vi "REFPROPdll_Test.vi"(8 "error in (no error)":errorcluster) -> (0 "error out":errorcluster, 3 "Passed?":bool)   [LabVIEW 2016]
panel:
  out "Inputs":T1
  out "Outputs":T2
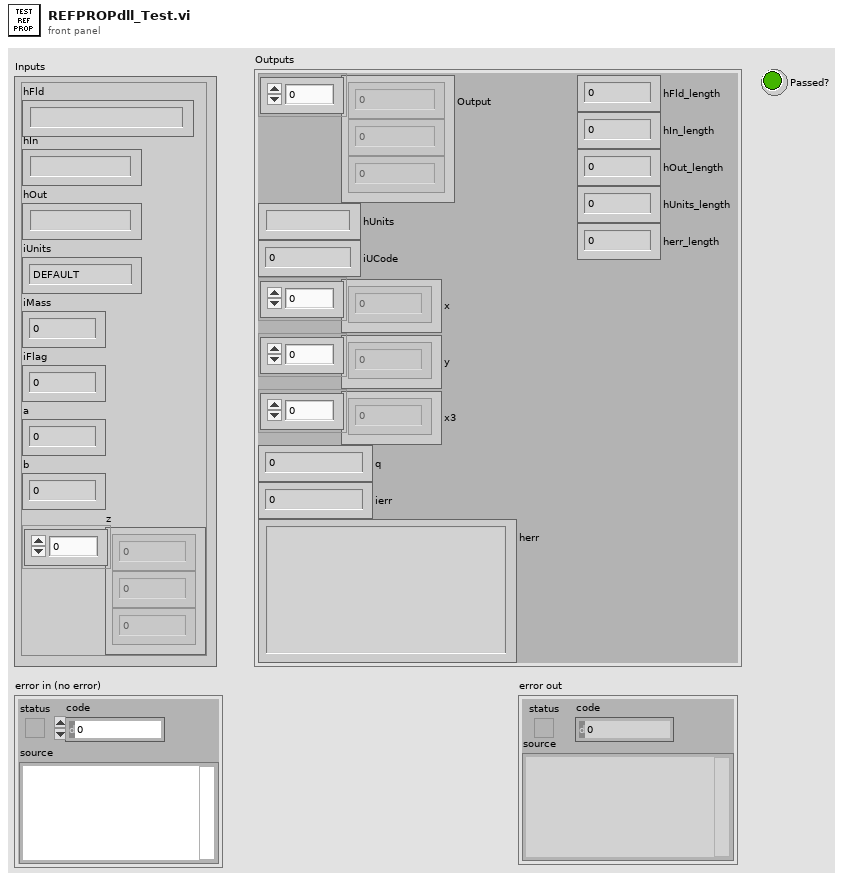
[diagram p1: front panel]
types:
  T1 = cluster{"hFld":string, "hIn":string, "hOut":string, "iUnits":enum32{"DEFAULT", "MOLE SI", "MASS SI", "SI WITH C"}, "iMass":i32, "iFlag":i32, "a":dbl, "b":dbl, "z":dbl[]}
  T2 = cluster{"Output":dbl[], "hUnits":string, "iUCode":i32, "x":dbl[], "y":dbl[], "x3":dbl[], "q":dbl, "ierr":i32, "herr":string, "hFld_length":i32, "hIn_length":i32, "hOut_length":i32, "hUnits_length":i32, "herr_length":i32}
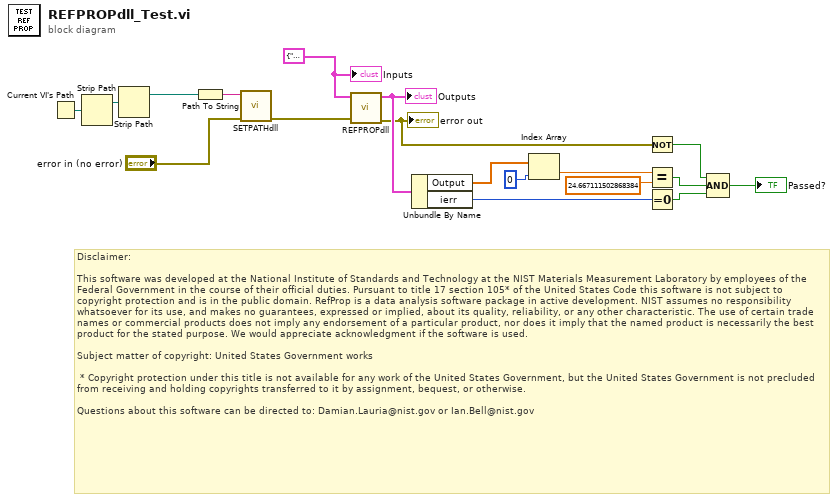
[diagram p0: block diagram]
diagram:
  w12 = T1 {"hFld"="Methane * Ethane", "hIn"="TQ", "hOut"="D", "iUnits"=enum."DEFAULT", "iMass"=0, "iFlag"=0, "a"=80.0, "b"=0.0, "z"=[0.4, 0.6]} ("Inputs")
  # "Disclaimer:\n\nThis software was developed at the National Institute of Standards and Technology at the NIST Materials Measurement Laboratory by employees of the Federal Government in the course of their official duties. Pursuant to title 17 section 105* of the United States Code this software is not subject to copyright protection and is in the public domain. RefProp is a data analysis software package in active development. NIST assumes no responsibility whatsoever for its use, and makes no guarantees, expressed or implied, about its quality, reliability, or any other characteristic. The use of certain trade names or commercial products does not imply any endorsement of a particular product, nor does it imply that the named product is necessarily the best product for the stated purpose. We would appreciate acknowledgment if the software is used.\n \nSubject matter of copyright: United States Government works\n  \n * Copyright protection under this title is not available for any work of the United States Government, but the United States Government is not precluded from receiving and holding copyrights transferred to it by assignment, bequest, or otherwise.\n\nQuestions about this software can be directed to: Damian.Lauria@nist.gov or Ian.Bell@nist.gov"
  n1 = Current VI's Path() -> (path=w18:path)
  n2 = Strip Path(path=w18) -> (stripped path=w17:path)  [unwired: 1 out]
  n3 = Strip Path(path=w17) -> (stripped path=w16:path)  [unwired: 1 out]
  n4 = Path To String(path=w16) -> (string=w15:string)
  n5 = call "SETPATHdll.vi"("error in (no error)"="error in (no error)", "hpath"=w15) -> ("error out"=w13:errorcluster)  [unwired: 7 in, 2 out]
  n6 = call "REFPROPdll.vi"("error in (no error)"=w13, "Inputs"=w12) -> ("error out"=w1:errorcluster, "Outputs"=w2:T2)  [unwired: 8 in]
  "Outputs" <- w2
  "error out" <- w1
  n7 = Unbundle By Name(w2) -> ("Output"=w10:dbl[], "ierr"=w11:i32)
  n8 = Index Array(array=w10, index=0) -> (element=w9:dbl)
  n9 = Not(x=w1) -> (.not. x?=w6:bool)
  n10 = Equal?(x=w9, y=24.667111502868384 ("element")) -> (x = y?=w5:bool)
  n11 = Equal To 0?(x=w11) -> (x = 0?=w4:bool)
  n12 = Compound Arithmetic op=AND(w6, w5, w4) -> (→"Passed?":bool)
  "Inputs" <- w12
